vi "Convert C to F.vi"(8 "error in (no error)":errorcluster, 9 "Container State":T2, 10 "Degrees Celsius":dbl, 11 "Display State In":T1) -> (0 "error out":errorcluster, 1 "Degrees Fahrenheit":dbl, 3 "Display State Out":T1)   [LabVIEW 2013, in "Simple Dual Mode Thermometer XControl.xctl"]
doc: "This VI handles the Convert C to F method as part of the Simple Dual Mode Thermometer XControl."
uses:
  Simple Dual Mode Thermometer XControl.xctl
  <vilib>/_xctls/Container State.ctl
  Simple Dual Mode Thermometer State.ctl
  <vilib>/_xctls/XControlSupport.lvlib
panel:
  # "Add controls and indicators that form the parameters of the method here and connect them to the connector pane. Do not delete the controls and indicators that are already connected.\n \nTo set up the parameters for this method, right click on this item in the Project Tree and select Configure Method..."
  # "This simple method converts degrees Celsius to degrees Fahrenheit."
  # "The State control is used for any variables that will affect the appearance or the data manipulation of the XControl. For the Simple DMT we only need to know if the data is being displayed as Fahrenheit."
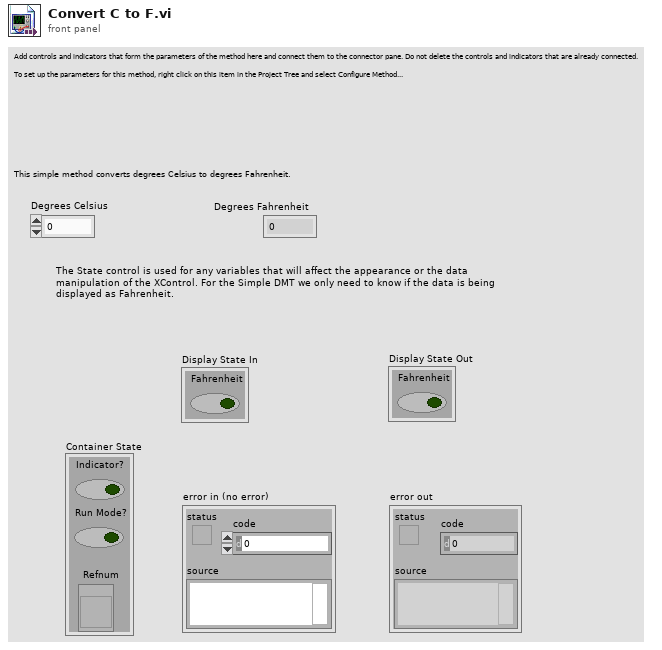
[diagram p1: front panel]
types:
  T1 = typedef "Simple Dual Mode Thermometer XControl.xctl/Simple Dual Mode Thermometer State.ctl" = cluster{"Fahrenheit":bool}
  T2 = typedef "XControlSupport.lvlib/Container State.ctl" = cluster{"Indicator?":bool, "Run Mode?":bool, " Refnum":refnum<vi>}
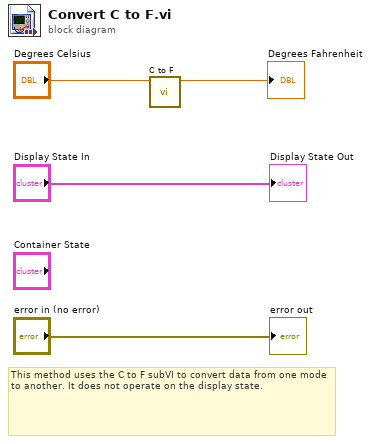
[diagram p0: block diagram]
diagram:
  # "This method uses the C to F subVI to convert data from one mode to another. It does not operate on the display state."
  n1 = call "C to F.vi"("Celsius"="Degrees Celsius") -> ("Fahrenheit"=→"Degrees Fahrenheit":dbl)  [unwired: 10 in]
  "Display State Out" <- "Display State In"
  "error out" <- "error in (no error)"
